vi "Item Outdent.vi"(0 "Tree Reference In":refnum<vi>, 2 "Outdent Item Tag (Current)":string, 5 "error in (no error)":errorcluster) -> (14 "Tree Reference Out":refnum<vi>, 19 "error out":errorcluster)   [LabVIEW 2011, in "VITesterUtilities.lvlib"]
doc: "Outdents the currently selected item or the input tag to the same indent level of its parent. Places in the topmost position of its siblings thus disrupting the order. If already at the most mature level in the tree, it moves it to the top of the structure."
uses:
  Libraries/VITesterUtilities.lvlib
panel:
  # "VI INPUTS"
  # "VI OUTPUTS"
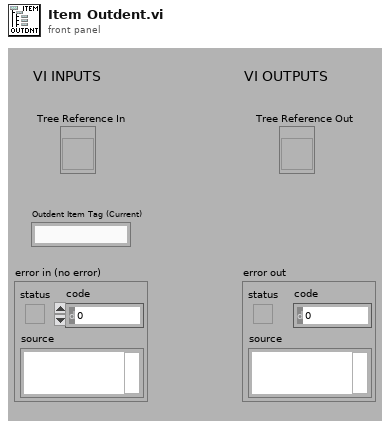
[diagram p1: front panel]
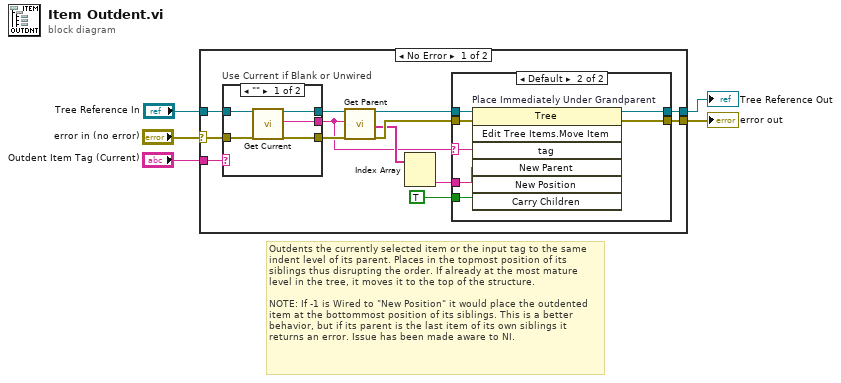
[diagram p0: block diagram]
diagram:
  # "Outdents the currently selected item or the input tag to the same indent level of its parent. Places in the topmost position of its siblings thus disrupting the order. If already at the most mature level in the tree, it moves it to the top of the structure.\n\nNOTE: If -1 is Wired to \"New Position\" it would place the outdented item at the bottommost position of its siblings. This is a better behavior, but if its parent is the last item of its own siblings it returns an error. Issue has been made aware to NI."
  n1 = case shown="No Error" "error in (no error)" {
    selector: "error in (no error)" -> [w10 w36]
    tunnel: "Tree Reference In" -> [w11 w37]
    tunnel: [w17 w37] -> w4
    tunnel: [w16 w36] -> w3
    tunnel: "Outdent Item Tag (Current)" -> [w9 _]
    frame No Error {
      n2 = case "Use Current if Blank or Unwired" shown="\"\"" w9 {
        selector: w9 -> [_ w33]
        tunnel: [w31 w35] -> w8
        tunnel: w11 -> [w32 w35]
        tunnel: [w30 w34] -> w7
        tunnel: w10 -> [w29 w34]
        tunnel: [w28 w33] -> w6
        frame "" {
          n3 = call "Get Current.vi"("Tree Reference In"=w32, "error in (no error)"=w29) -> ("Tree Reference Out"=w31:refnum<vi>, "Current Tag"=w28:string, "error out"=w30:errorcluster)  [unwired: 14 in, 1 out]
        }
        frame Default {
        }
      }
      n4 = call "Get Parent.vi"("Tree Reference In"=w8, "Child Tag (Current)"=w6, "error in (no error)"=w7) -> ("Tree Reference Out"=w13:refnum<vi>, "Parents Tags"=w15:string[], "error out"=w18:errorcluster)  [unwired: 13 in, 1 out]
      n5 = Index Array(array=w15) -> (element #2=w12:string)  [unwired: 2 in, 1 out]
      n6 = case shown="Default" w6 {
        selector: w6 -> [_ w21]
        tunnel: w18 -> [w19 w27]
        tunnel: [w20 w26] -> w17
        tunnel: [w19 w25] -> w16
        tunnel: TRUE ("Carry Children") -> [_ w24]
        tunnel: w13 -> [w20 w23]
        tunnel: w12 -> [_ w22]
        frame "" {
        }
        frame Default {
          n7 = invoke on="Place Immediately Under Grandparent" class="Tree" method="Edit Tree Items.Move Item"(reference=w23, error in=w27, "tag"=w21, "New Parent"=w22, "Carry Children"=w24) -> (reference out=w26:refnum<vi>, error out=w25:errorcluster)  [unwired: 2 in, 5 out]
        }
      }
    }
    frame Error {
    }
  }
  "Tree Reference Out" <- w4
  "error out" <- w3
